vi "Simulated Starter Kit 2.0 Roaming.vi"() -> ()   [LabVIEW 2012]
doc: "This VI demonstrates how to control a simulated Robotics Starter Kit 2.0 robot. With a few modifications, you can deploy this VI to the Single-Board RIO 9632 on a real robot, and it runs on the real-time controller. For more information about how to modify this VI so you can deploy it to real hardware, refer to the <B>Robotics Module>>Simulating Mobile Robots</B> book on the <B>Contents</B> tab of the LabVIEW Help."
uses:
  <vilib>/Platform/TimedLoop/XDataNode/timing_clust.ctl
  <vilib>/Platform/TimedLoop/XDataNode/nitl_modes.ctl
  <vilib>/Platform/TimedLoop/XDataNode/wakeup.ctl
  <vilib>/robotics/Starter Kit/2.0/Sim Host Interface/NI_Robotics_Starter Kit Host_Sim_2.0.lvclass
  <vilib>/Utility/AngleManip/Degrees to Radians (Scalar DBL).vi
  <vilib>/robotics/Steering/Steering Frame/Apply Steering Frame Velocity to Motors.vi
  <vilib>/Platform/TimedLoop/XDataNode/XDataNode.xnode
  <vilib>/Platform/TimedLoop/XDataNode/XDNodeRunTimeDep.lvlib
  <vilib>/Utility/AngleManip/NI_AngleManipulation.lvlib
  <vilib>/robotics/Utilities/Scan Angles/NI_Robotics_Scan Angles.lvlib
  <vilib>/robotics/Steering/Steering Frame/NI_Robotics_Steering Frame.lvclass
  <vilib>/robotics/Starter Kit/Host Interface/NI_Robotics_Starter Kit Host.lvclass
  <vilib>/robotics/Starter Kit/2.0/NI_Robotics_Starter Kit Host_2.0.lvlib
  <vilib>/robotics/Simulator/NI_Robotics_Simulator.lvlib
panel:
  out "Sensor Data":cluster{"angles (deg)":dbl[], "distances":dbl[]}(graph)
  in  "stop":bool
  # "This VI demonstrates how to control a simulated Robotics Starter Kit 2.0 robot.\n\nRun this VI to launch the simulation.  The simulated environment is displayed in a separate window.  The graph displays the range data acquired by the simulated ultrasonic sensor on the robot.  Click the STOP button to end the simulation."
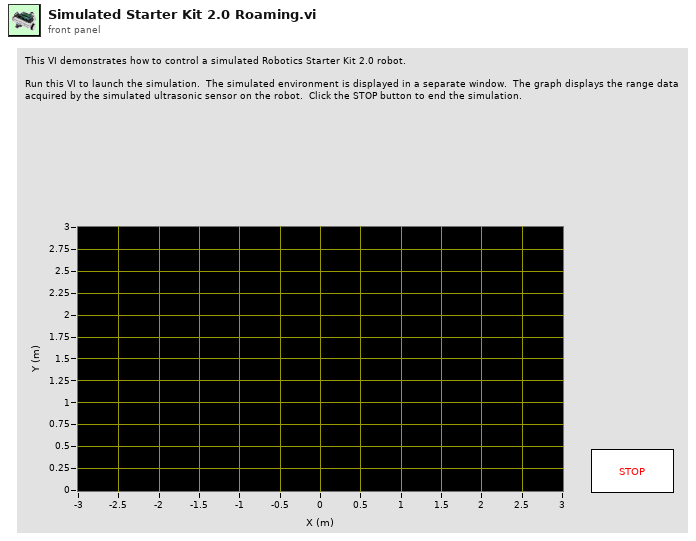
[diagram p1: front panel]
types:
  T1 = typedef "XDNodeRunTimeDep.lvlib/timing_clust.ctl" = cluster{"Expected End [f-1]":u64, "Actual End [f-1]":u64, "Finished Late? [f-1]":bool, "Expected End [i-1]":u64, "Actual End [i-1]":u64, "Finished Late? [i-1]":bool, "Expected Start [i]":u64, "Actual Start [i]":u64, "Expected Start [f]":u64, "Actual Start [f]":u64, "Source Name":string, "Structure Name":string, "Period":i64, "Deadline":i64, "Offset":i64, "Start":i64, "Priority":i32, "Timeout":i32, "Mode":T2, "Wakeup Reason":T3, "Error":errorcluster, "Source Type":string, "Secondary Source Type":string, "Global End Time":u64, "Global Start Time":u64, "Frame Duration":u64, "Iteration Duration":u64, "Assigned CPU":i32, "I/O Scan Engine Mode":u32}
  T2 = typedef "XDNodeRunTimeDep.lvlib/nitl_modes.ctl" = enum32{"No Change", "Process missed periods, maintain original phase", "Discard missed periods, maintain original phase", "Process missed periods, ignore original phase", "Discard missed periods, ignore original phase"}
  T3 = typedef "XDNodeRunTimeDep.lvlib/wakeup.ctl" = enum32{"Normal", "Aborted", "Asynchronous wakeup", "Timing source error", "Timed loop error", "Timeout"}
  T4 = typedef "NI_Robotics_Scan Angles.lvlib/Scan Angle Data.ctl" = cluster{"angles":dbl[], "distances":dbl[], "current index":i32, "previous index":i32}
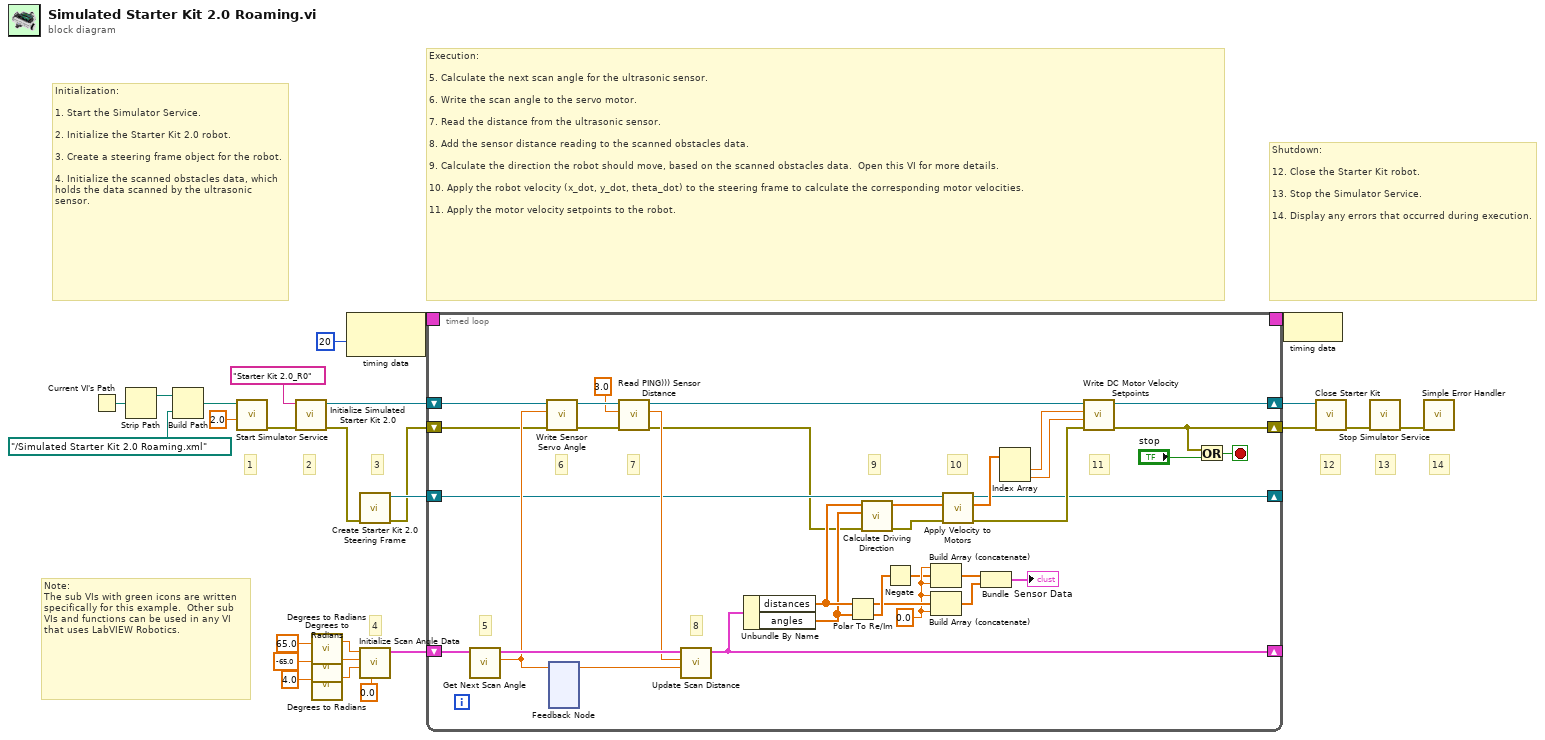
[diagram p0: block diagram]
diagram:
  # "14"
  # "13"
  # "12"
  # "Execution:\n\n5. Calculate the next scan angle for the ultrasonic sensor.\n\n6. Write the scan angle to the servo motor.\n\n7. Read the distance from the ultrasonic sensor.\n\n8. Add the sensor distance reading to the scanned obstacles data.\n\n9. Calculate the direction the robot should move, based on the scanned obstacles data.  Open this VI for more details.\n\n10. Apply the robot velocity (x_dot, y_dot, theta_dot) to the steering frame to calculate the corresponding motor velocities.\n\n11. Apply the motor velocity setpoints to the robot."
  # "1"
  # "Shutdown:\n\n12. Close the Starter Kit robot.\n\n13. Stop the Simulator Service.\n\n14. Display any errors that occurred during execution."
  # "Note:\nThe sub VIs with green icons are written specifically for this example.  Other sub VIs and functions can be used in any VI that uses LabVIEW Robotics."
  # "2"
  # "3"
  # "4"
  # "Initialization:\n\n1. Start the Simulator Service.\n\n2. Initialize the Starter Kit 2.0 robot.\n\n3. Create a steering frame object for the robot.\n\n4. Initialize the scanned obstacles data, which holds the data scanned by the ultrasonic sensor."
  n1 = Current VI's Path() -> (path=w25:path)
  n2 = Strip Path(path=w25) -> (stripped path=w26:path)  [unwired: 1 out]
  n3 = Build Path(base path=w26, name or relative path=path "../Simulated Starter Kit 2.0 Roaming.xml" ("Simulation Manifest File")) -> (appended path=w5:path)
  n4 = call <vilib>:"Start Simulator Service.vi"("step size (ms)"=2.0, "manifest file"=w5) -> ("error out"=w3:errorcluster)  [unwired: 9 in]
  n5 = call <vilib>:"Initialize Simulated Starter Kit 2.0.vi"("error in (no error)"=w3, "robot ID"="Starter Kit 2.0_R0") -> ("error out"=w19:errorcluster, "simulated starter kit host 2.0 out"=w20:refnum<class "NI_Robotics_Starter Kit Host_Sim_2.0.lvclass">)  [unwired: 8 in]
  n6 = call-poly <vilib>:"Degrees to Radians.vi"("angle (deg)"=65.0 ("max angle")) -> ("angle (rad)"=w15:dbl)  [unwired: 2 in]
  n7 = call-poly <vilib>:"Degrees to Radians.vi"("angle (deg)"=-65.0 ("min angle")) -> ("angle (rad)"=w11:dbl)  [unwired: 2 in]
  n8 = call-poly <vilib>:"Degrees to Radians.vi"("angle (deg)"=4.0 ("scan angle")) -> ("angle (rad)"=w12:dbl)  [unwired: 2 in]
  n9 = node-c288(i64 20 ("Period")) -> (w24:T1)
  n10 = call <vilib>:"Create Starter Kit 2.0 Steering Frame.vi"("error in (no error)"=w19) -> ("error out"=w9:errorcluster, "starter kit differential steering frame"=w21:refnum<class "NI_Robotics_Differential Steering Frame.lvclass">)  [unwired: 9 in]
  n11 = call <vilib>:"Initialize Scan Angle Data.vi"("initial angle (0)"=0.0, "scan angle"=w12, "min angle"=w11, "max angle"=w15) -> ("scan angles"=w10:T4)  [unwired: 6 in, 1 out]
  n12 = timed-loop {
    shift-right: [w41] -> w18
    shift-left: w20 -> [w46]
    shift-right: [w27] -> w17
    shift-left: w9 -> [w43]
    shift-right: [w44] -> _
    shift-left: w21 -> [w45]
    timing: w24 -> [_]
    timing-out: [_] -> w23
    shift-right: [w40] -> _
    shift-left: w10 -> [w47]
    stop <- w42 stop-if-true
    w36 = 0.0 ("element")
    # "7"
    # "6"
    # "11"
    # "10"
    # "9"
    # "8"
    # "5"
    n13 = call <vilib>:"Get Next Scan Angle.vi"("scan angles in"=w47) -> ("new angle"=w56:dbl, "scan angles out"=w59:T4)  [unwired: 9 in]
    n14 = call <vilib>:"Write Sensor Servo Angle.vi"("error in (no error)"=w43, "ccw servo angle (rad)"=w56, "starter kit host in"=w46) -> ("error out"=w53:errorcluster, "starter kit host out"=w54:refnum<class "NI_Robotics_Starter Kit Host_Sim_2.0.lvclass">)  [unwired: 7 in]
    n15 = feedback #1() -> (w58:dbl)  [unwired: 1 in]
    n16 = feedback-in #1(w56) -> ()
    n17 = call <vilib>:"Read PING))) Sensor Distance.vi"("error in (no error)"=w53, "default distance (NaN)"=3.0, "starter kit host in"=w54) -> ("error out"=w29:errorcluster, "distance (m)"=w55:dbl, "starter kit host out"=w52:refnum<class "NI_Robotics_Starter Kit Host_Sim_2.0.lvclass">)  [unwired: 5 in, 1 out]
    n18 = call <vilib>:"Update Scan Distance.vi"("scan angle"=w58, "new scan distance"=w55, "scan angles in"=w59) -> ("scan angles out"=w40:T4)  [unwired: 8 in]
    n19 = Unbundle By Name(w40) -> ("distances"=w32:dbl[], "angles"=w30:dbl[])
    n20 = Polar To Re/Im(2:w30, 3:w32) -> (0:w39:dbl[], 1:w38:dbl[])
    n21 = call "Calculate Driving Direction.vi"("error in (no error)"=w29, "obstacle angles (rad)"=w30, "obstacle distances (m)"=w32) -> ("error out"=w28:errorcluster, "steering frame velocity"=w31:dbl[])  [unwired: 7 in]
    n22 = Negate(x=w39) -> (-x=w34:dbl[])
    n23 = Build Array (concatenate)(w36, w34, w36) -> (w35:dbl[])
    n24 = Build Array (concatenate)(w36, w38, w36) -> (w37:dbl[])
    n25 = call-poly <vilib>:"Apply Velocity to Motors.vi"("error in (no error)"=w28, "steering frame velocity"=w31, "steering frame in"=w45) -> ("error out"=w51:errorcluster, "ccw motor velocity setpoints"=w57:dbl[], "steering frame out"=w44:refnum<class "NI_Robotics_Differential Steering Frame.lvclass">)  [unwired: 4 in, 2 out]
    n26 = Bundle(w35, w37) -> (→"Sensor Data":cluster{dbl[], dbl[]})  [unwired: 1 in]
    n27 = Index Array(array=w57) -> (element #1=w50:dbl, element #2=w49:dbl)  [unwired: 2 in]
    n28 = call <vilib>:"Write DC Motor Velocity Setpoints.vi"("error in (no error)"=w51, "right motor ccw velocity (rad/s)"=w49, "left motor ccw velocity (rad/s)"=w50, "starter kit host in"=w52) -> ("error out"=w27:errorcluster, "starter kit host out"=w41:refnum<class "NI_Robotics_Starter Kit Host_Sim_2.0.lvclass">)  [unwired: 6 in]
    n29 = Or(x=w27, y="stop") -> (x .or. y?=w42:bool)
  }
  n30 = node-c288(w23) -> ()
  n31 = call-dynamic "Close Starter Kit.vi"("error in (no error)"=w17, "starter kit host in"=w18) -> ("error out"=w2:errorcluster)  [unwired: 9 in]
  n32 = call <vilib>:"Stop Simulator Service.vi"("error in (no error)"=w2) -> ("error out"=w1:errorcluster)  [unwired: 10 in]
  n33 = call <vilib>:"Simple Error Handler.vi"("error in (no error)"=w1) -> ()  [unwired: 4 in, 5 out]
